vi "Camera Tester.vi"() -> ()   [LabVIEW 2020]
uses:
  <vilib>/userdefined/High Color/IMAQdx.ctl
  <vilib>/vision/driver/NI_Vision_Acquisition_Software.lvlib
panel:
  in  "stop":bool
  out "Image":T1(plugin-control)
  out "Acquired Frames/s":dbl
  out "Distance (calibrated)":sgl format="%.2f"
  in  "Session In":T2
  in  "Color Plane":i32(ring)=1 items=["Red", "Green", "Blue", "Hue", "Saturation", "Luminance", "Value", "Intensity"]
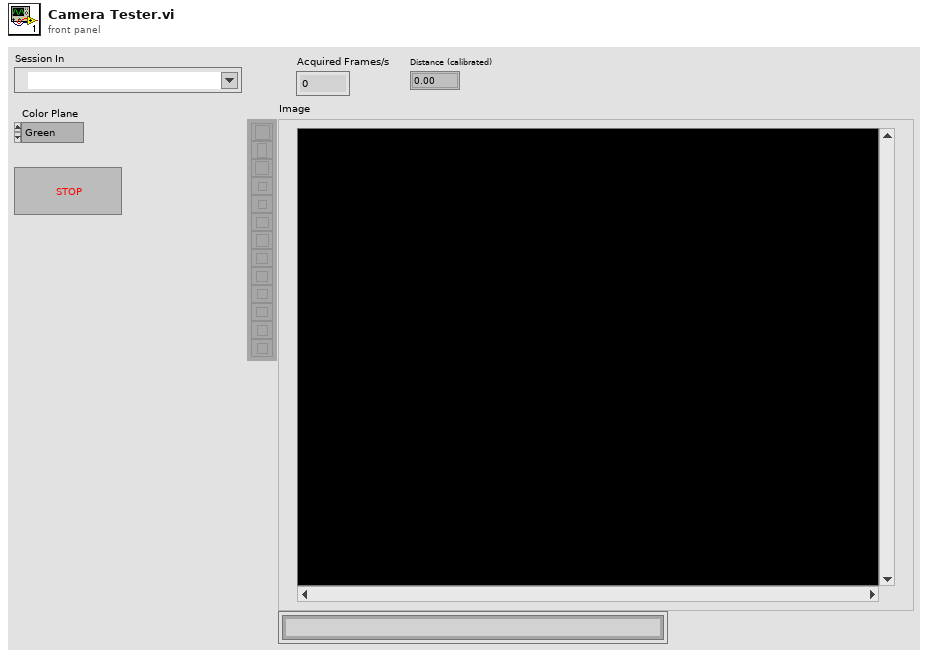
[diagram p1: front panel]
types:
  T1 = typedef "IMAQ Image.ctl" = refnum<image>
  T2 = typedef "IMAQdx.ctl" = refnum<k21>
  T3 = typedef "Image Type" = u32
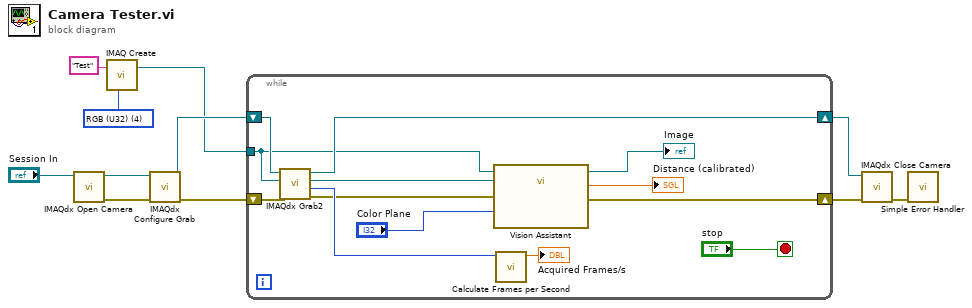
[diagram p0: block diagram]
diagram:
  w8 = T3 4 items=["Grayscale (U8)", "Grayscale (I16)", "Grayscale (SGL)", "Complex (CSG)", "RGB (U32)", "HSL (U32)", "RGB (U64)", "Grayscale (U16)"] ("Image Type")
  n1 = call <vilib>:"IMAQdx Open Camera.vi"("Session In"="Session In") -> ("error out"=w11:errorcluster, "Session Out"=w10:T2)  [unwired: 9 in]
  n2 = call "IMAQ Create"("Image Name"="Test", "Image Type"=w8) -> ("New Image"=w3:T1)  [unwired: 3 in, 1 out]
  n3 = call <vilib>:"IMAQdx Configure Grab.vi"("error in"=w11, "Session In"=w10) -> ("error out"=w7:errorcluster, "Session Out"=w6:T2)  [unwired: 8 in]
  n4 = while {
    tunnel: w3 -> [w16]
    shift-right: [w13] -> w2
    shift-left: w7 -> [w22]
    shift-right: [w20] -> w4
    shift-left: w6 -> [w21]
    stop <- "stop" stop-if-true
    n5 = call <vilib>:"IMAQdx Grab2.vi"("error in"=w22, "Image In"=w16, "Session In"=w21) -> ("error out"=w15:errorcluster, "Buffer Number Out"=w24:u32, "Image Out"=w17:T1, "Session Out"=w20:T2)  [unwired: 5 in]
    n6 = call "Vision Assistant"("Image In"=w16, "Image Dst"=w17, "Color Plane (Color Plane Extraction 1)"="Color Plane", "error in"=w15) -> ("Image Out"=→"Image":T1, "Distance (calibrated) (Clamp (Rake) 1)"=→"Distance (calibrated)":sgl, "error out"=w13:errorcluster)  [unwired: 21 in]
    n7 = call <vilib>:"Calculate Frames per Second.vi"("Buffer Number"=w24) -> ("Acquired Frames/s"=→"Acquired Frames/s":dbl)  [unwired: 8 in, 2 out]
  }
  n8 = call <vilib>:"IMAQdx Close Camera.vi"("error in"=w2, "Session In"=w4) -> ("error out"=w1:errorcluster)  [unwired: 9 in]
  n9 = call <vilib>:"Simple Error Handler.vi"("error in (no error)"=w1) -> ()  [unwired: 4 in, 5 out]
